vi "BDSCTRL_Read_Configuration_Settings_File.vi"(0 "configuration file path":path, 5 "error in \n(no error)":errorcluster) -> (6 "Channels Cluster":T7={"TX1"=TRUE, "TX2"=TRUE, "TX3"=FALSE, "TX4"=FALSE, "TXx3"=TRUE, "TXx4"=TRUE, "RX1"=FALSE, "RX2"=FALSE, "RX3"=FALSE, "RX4"=FALSE, "RXx3"=FALSE, "RXx4"=FALSE, "Tx"=TRUE, "Rx"=FALSE}, 7 "Set Beam Settings Cluster":T2, 8 "Beam Rotation":string[][](table)=[["1"], ["1"], ["1"], ["1"], ["1"], ["1"], ["2"], ["2"], ["2"], ["2"], ["2"], ["2"]], 9 "DMA Settings Cluster":T1, 10 "Target Devices Settings Cluster":T4={"Target Devices"={"P1 Cluster"={"P1_D1"=TRUE, "P1_D2"=TRUE, "P1_D3"=TRUE, "P1_D4"=TRUE, "P1_D5"=TRUE, "P1_D6"=TRUE, "P1_D7"=TRUE, "P1_D8"=TRUE, "P1_D9"=TRUE, "P1_D10"=TRUE, "P1_D11"=TRUE, "P1_D12"=TRUE, "P1_D13"=TRUE, "P1_D14"=TRUE, "P1_D15"=TRUE, "P1_D16"=TRUE, "P1_D17"=TRUE, "P1_D18"=TRUE, "P1_D19"=TRUE, "P1_D20"=TRUE, "P1_D21"=TRUE, "P1_D22"=TRUE, "P1_D23"=TRUE, "P1_D24"=TRUE}, "P2 Cluster"={"P2_D1"=TRUE, "P2_D2"=TRUE, "P2_D3"=TRUE, "P2_D4"=TRUE, "P2_D5"=TRUE, "P2_D6"=TRUE, "P2_D7"=TRUE, "P2_D8"=TRUE, "P2_D9"=TRUE, "P2_D10"=TRUE, "P2_D11"=TRUE, "P2_D12"=TRUE, "P2_D13"=TRUE, "P2_D14"=TRUE, "P2_D15"=TRUE, "P2_D16"=TRUE, "P2_D17"=TRUE, "P2_D18"=TRUE, "P2_D19"=TRUE, "P2_D20"=TRUE, "P2_D21"=TRUE, "P2_D22"=TRUE, "P2_D23"=TRUE, "P2_D24"=TRUE}}, "Target String"="{1:24,1:24,[],[]}"}, 11 "MB-CFR Settings Cluster":T5, 12 "RF Parameters Settings Cluster":T3={"Tx RF \nFrequency"=2132.5, "RF Bandwidth \n(MHz)"=0, "Tx VGA"=[], "Rx VGA"=[]}, 14 "BDSCTRL Connection Settings":T9={"Panel IP Address"="10.1.11.247", "Melvitron IP Address"="COM12", "EXA IP Address"="10.1.11.123", "MXG IP Address"="10.1.11.122"}, 15 "Test Setup Settings":T8={"IF Calibration File"=path "IFCalExample.csv", "Beam Lookup Table"=path "BeamLookupTableExample.csv", "Test Environment"=enum."Melvitron", "Panel Mode"=enum."CPRI", "Calibration Mode"=0, "Panel Type"=0, "Band"=0, "Tile"=0, "API Drop"=0} {"API Drop" items=["MAY", "JUNE"]; "Tile" items=["HP-C", "HP-B3"]; "Band" items=["AWS", "PCS-A", "PCS-G"]; "Panel Type" items=["Half", "Full", "Quarter"]; "Calibration Mode" items=["Manual", "SemiAuto", "Auto"]}, 16 "Panel Action Sequence":T6[](array[typedef]) items=["Panel Init", "RF Calibration", "Rotate Beam", "Set RF Frequency", "Initial Calibrations", "Channel Enable", "IF Calibration", "Sense Power", "Measure Temperature", "Set RF Power Level", "Run DMA", "Set RF Bandwidth", "Set CFR", "Set Beam"], 19 "error out":errorcluster)   [LabVIEW 2016]
doc: "Illustrates how to read a configuration settings file.\n\nInstructions:\nRun Write Configuration Settings File.vi, located in the file\\config.llb. Then run this VI and select the appropriate configuration settings file to load."
uses:
  BDSCTRL_Controls/BDSCTRL_Panel_Action_List.ctl
  <vilib>/Utility/config.llb/Read Key (String).vi
  <vilib>/Utility/config.llb/Read Key (Path).vi
  <vilib>/Utility/config.llb/Read Key (U32).vi
  <vilib>/Utility/config.llb/Read Key (Boolean).vi
  <vilib>/Utility/config.llb/Read Key (Double).vi
  <vilib>/Utility/config.llb/Read Key (I32).vi
  <vilib>/Utility/config.llb/NI_LVConfig.lvlib
panel:
  out "Instrument Mode Cluster":T10
  out "Array Indexing":string[](array[string])=["A", "B", "C", "D", "E", "F"]
  out "Test Config Size":i32
  out "Test Array Size":i32
  out "Test Array":T11(array[cluster])=[{"Test Module"=0, "Select"=TRUE, "Configure\nParameters"=FALSE}, {"Test Module"=0, "Select"=FALSE, "Configure\nParameters"=FALSE}, {"Test Module"=0, "Select"=FALSE, "Configure\nParameters"=FALSE}, {"Test Module"=0, "Select"=FALSE, "Configure\nParameters"=FALSE}, {"Test Module"=0, "Select"=FALSE, "Configure\nParameters"=FALSE}, {"Test Module"=0, "Select"=FALSE, "Configure\nParameters"=FALSE}, {"Test Module"=0, "Select"=FALSE, "Configure\nParameters"=FALSE}, {"Test Module"=0, "Select"=FALSE, "Configure\nParameters"=FALSE}, {"Test Module"=0, "Select"=FALSE, "Configure\nParameters"=FALSE}, {"Test Module"=0, "Select"=FALSE, "Configure\nParameters"=FALSE}, {"Test Module"=0, "Select"=FALSE, "Configure\nParameters"=FALSE}, {"Test Module"=0, "Select"=FALSE, "Configure\nParameters"=FALSE}, {"Test Module"=0, "Select"=FALSE, "Configure\nParameters"=FALSE}, {"Test Module"=0, "Select"=FALSE, "Configure\nParameters"=FALSE}, {"Test Module"=0, "Select"=FALSE, "Configure\nParameters"=FALSE}, {"Test Module"=0, "Select"=FALSE, "Configure\nParameters"=FALSE}, {"Test Module"=0, "Select"=FALSE, "Configure\nParameters"=FALSE}, {"Test Module"=0, "Select"=FALSE, "Configure\nParameters"=FALSE}, {"Test Module"=0, "Select"=FALSE, "Configure\nParameters"=FALSE}, {"Test Module"=0, "Select"=FALSE, "Configure\nParameters"=FALSE}] {"Test Module" items=["::Select_a_module::", "Dynamic_Range", "EVM_FreqErr_OutputPower_GainFlatness", "RSSI"]}
  # "DMA"
  # "Set Beam"
  # "RF Parameters"
  # "P2"
  # "P1"
  # "MB-CFR"
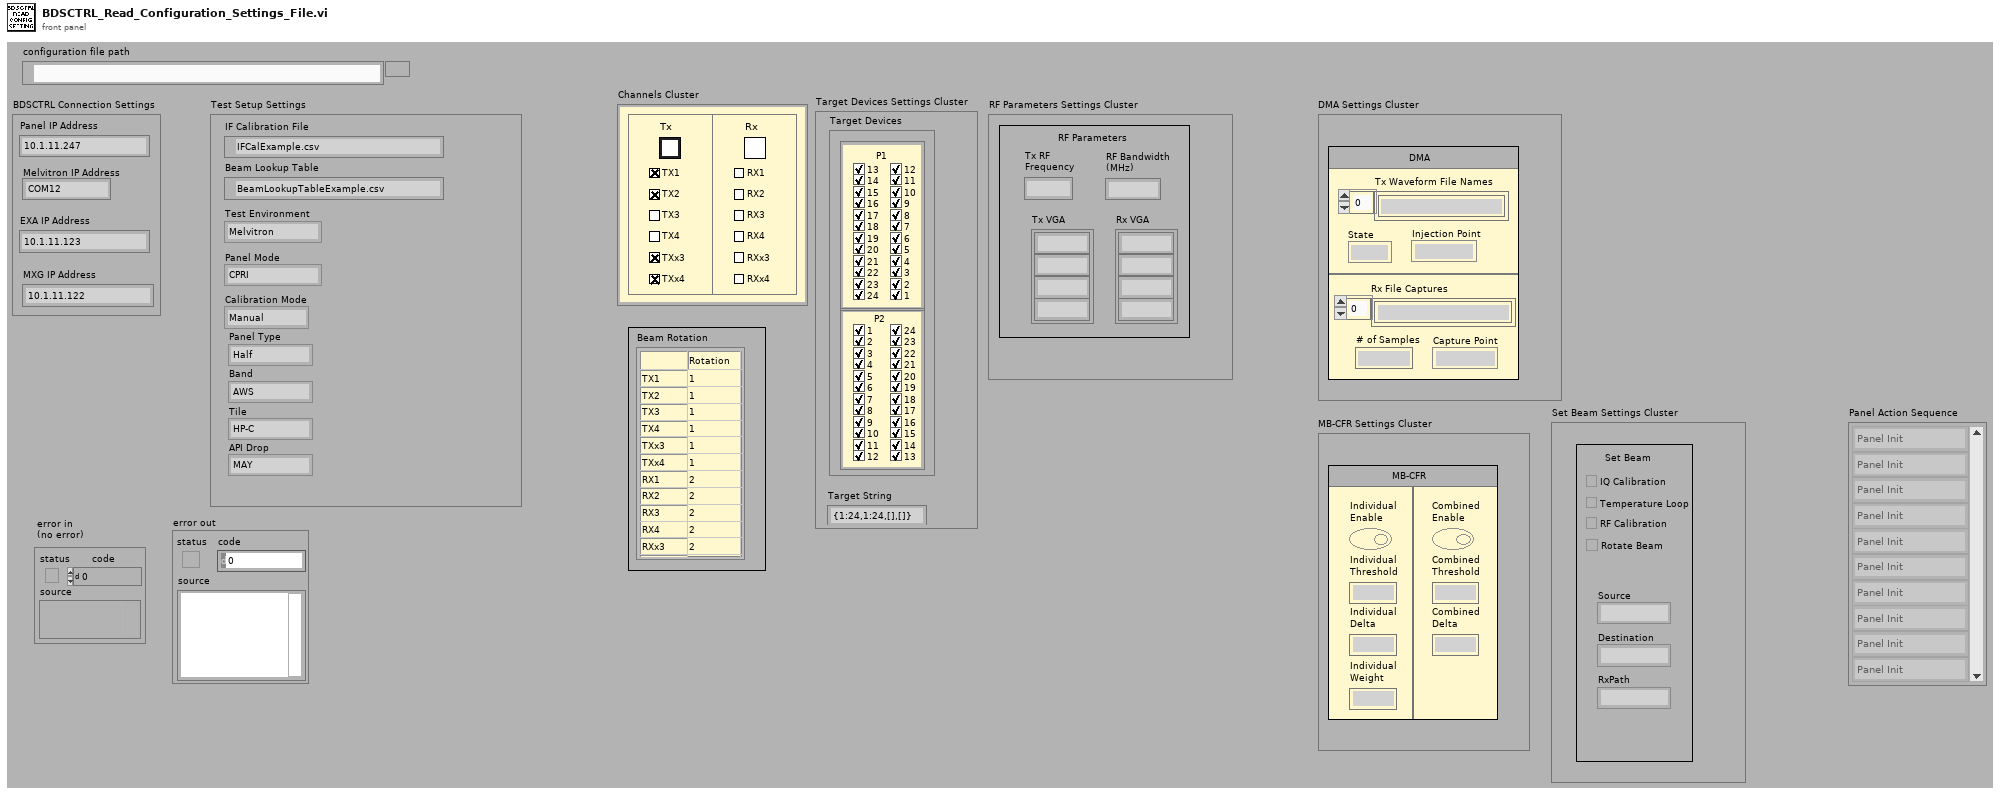
[diagram p1: front panel]
types:
  T1 = cluster{"Tx Waveform File Names":string[], "State":enum16{"Start", "Stop"}, "Injection Point":enum16{"MEM_DAC", "MEM_DUC"}, "Rx File Captures":string[], "# of Samples":i32, "Capture Point":enum16{"MEM_ADC", "MEM_DDC"}}
  T2 = cluster{"IQ Calibration":bool, "Temperature Loop":bool, "RF Calibration":bool, "Rotate Beam":bool, "Source":enum16{"CPRI", "CAL", "MEM_DAC", "MEM_DUC", "EXT"}, "Destination":enum16{"CPRI", "EXT", "MEM_ADC", "MEM_DDC"}, "RxPath":enum16{"DIRECT", "MIXER"}}
  T3 = cluster{"Tx RF \nFrequency":dbl, "RF Bandwidth \n(MHz)":i32, "Tx VGA":i32[], "Rx VGA":i32[]}
  T4 = cluster{"Target Devices":cluster{"P1 Cluster":cluster{"P1_D1":bool, "P1_D2":bool, "P1_D3":bool, "P1_D4":bool, "P1_D5":bool, "P1_D6":bool, "P1_D7":bool, "P1_D8":bool, "P1_D9":bool, "P1_D10":bool, "P1_D11":bool, "P1_D12":bool, "P1_D13":bool, "P1_D14":bool, "P1_D15":bool, "P1_D16":bool, "P1_D17":bool, "P1_D18":bool, "P1_D19":bool, "P1_D20":bool, "P1_D21":bool, "P1_D22":bool, "P1_D23":bool, "P1_D24":bool}, "P2 Cluster":cluster{"P2_D1":bool, "P2_D2":bool, "P2_D3":bool, "P2_D4":bool, "P2_D5":bool, "P2_D6":bool, "P2_D7":bool, "P2_D8":bool, "P2_D9":bool, "P2_D10":bool, "P2_D11":bool, "P2_D12":bool, "P2_D13":bool, "P2_D14":bool, "P2_D15":bool, "P2_D16":bool, "P2_D17":bool, "P2_D18":bool, "P2_D19":bool, "P2_D20":bool, "P2_D21":bool, "P2_D22":bool, "P2_D23":bool, "P2_D24":bool}}, "Target String":string}
  T5 = cluster{"Individual\nEnable":bool, "Individual\nThreshold":dbl, "Individual\nDelta":dbl, "Individual\nWeight":dbl, "Combined\nEnable":bool, "Combined\nThreshold":dbl, "Combined\nDelta":dbl}
  T6 = typedef "BDSCTRL_Panel_Action_List.ctl" = u16
  T7 = cluster{"TX1":bool, "TX2":bool, "TX3":bool, "TX4":bool, "TXx3":bool, "TXx4":bool, "RX1":bool, "RX2":bool, "RX3":bool, "RX4":bool, "RXx3":bool, "RXx4":bool, "Tx":bool, "Rx":bool}
  T8 = cluster{"IF Calibration File":path, "Beam Lookup Table":path, "Test Environment":enum16{"Melvitron", "Spider", "Marinotron"}, "Panel Mode":enum16{"CPRI", "UpDnCnv"}, "Calibration Mode":u16, "Panel Type":u16, "Band":u16, "Tile":u16, "API Drop":u16}
  T9 = cluster{"Panel IP Address":string, "Melvitron IP Address":string, "EXA IP Address":string, "MXG IP Address":string}
  T10 = cluster{"MXA Connection":cluster{"MXA":refnum<visa-resource-name>, "Entry Mode":enum16{"VISA", "IP Address"}}, "MXG1 Connection":cluster{"MXG 1":refnum<visa-resource-name>, "Entry Mode":enum16{"VISA", "IP Address"}}, "MXG2 Connection":cluster{"MXG 2":refnum<visa-resource-name>, "Entry Mode":enum16{"VISA", "IP Address"}}, "MXG3 Connection":cluster{"MXG 3":refnum<visa-resource-name>, "Entry Mode":enum16{"VISA", "IP Address"}}, "ENA Connection":cluster{"ENA":refnum<visa-resource-name>, "Entry Mode":enum16{"VISA", "IP Address"}}}
  T11 = cluster{"Test Module":u16, "Select":bool, "Configure\nParameters":bool}[]
  T12 = typedef "NI_LVConfig.lvlib/Config Data RefNum.ctl" = refnum<k1>
  T13 = cluster{"value":i32, i32[], "value":string, "value":bool, "value":i32, "value":path, "value":path, dbl[][], dbl[][]}
  T14 = cluster{cluster{"value":string, "value":i32}, cluster{"value":string, "value":i32}, cluster{"value":string, "value":i32}, cluster{"value":string, "value":i32}, cluster{"value":string, "value":i32}}
  T15 = cluster{"value":string, "value":string, "value":string, "value":string}
  T16 = cluster{"value":path, "value":path, "value":u32, "value":u32, "value":u32, "value":u32, "value":u32, "value":u32, "value":u32}
  T17 = cluster{"[0]":bool, "[1]":bool, "[2]":bool, "[3]":bool, "[4]":bool, "[5]":bool, "[6]":bool, "[7]":bool, "[8]":bool, "[9]":bool, "[10]":bool, "[11]":bool, "[12]":bool, "[13]":bool}
  T18 = cluster{"[0]":bool, "[1]":bool, "[2]":bool, "[3]":bool, "[4]":bool, "[5]":bool, "[6]":bool, "[7]":bool, "[8]":bool, "[9]":bool, "[10]":bool, "[11]":bool, "[12]":bool, "[13]":bool, "[14]":bool, "[15]":bool, "[16]":bool, "[17]":bool, "[18]":bool, "[19]":bool, "[20]":bool, "[21]":bool, "[22]":bool, "[23]":bool}
  T19 = cluster{"[0]":cluster{"[0]":bool, "[1]":bool, "[2]":bool, "[3]":bool, "[4]":bool, "[5]":bool, "[6]":bool, "[7]":bool, "[8]":bool, "[9]":bool, "[10]":bool, "[11]":bool, "[12]":bool, "[13]":bool, "[14]":bool, "[15]":bool, "[16]":bool, "[17]":bool, "[18]":bool, "[19]":bool, "[20]":bool, "[21]":bool, "[22]":bool, "[23]":bool}, "[1]":cluster{"[0]":bool, "[1]":bool, "[2]":bool, "[3]":bool, "[4]":bool, "[5]":bool, "[6]":bool, "[7]":bool, "[8]":bool, "[9]":bool, "[10]":bool, "[11]":bool, "[12]":bool, "[13]":bool, "[14]":bool, "[15]":bool, "[16]":bool, "[17]":bool, "[18]":bool, "[19]":bool, "[20]":bool, "[21]":bool, "[22]":bool, "[23]":bool}}
  T20 = cluster{cluster{"[0]":cluster{"[0]":bool, "[1]":bool, "[2]":bool, "[3]":bool, "[4]":bool, "[5]":bool, "[6]":bool, "[7]":bool, "[8]":bool, "[9]":bool, "[10]":bool, "[11]":bool, "[12]":bool, "[13]":bool, "[14]":bool, "[15]":bool, "[16]":bool, "[17]":bool, "[18]":bool, "[19]":bool, "[20]":bool, "[21]":bool, "[22]":bool, "[23]":bool}, "[1]":cluster{"[0]":bool, "[1]":bool, "[2]":bool, "[3]":bool, "[4]":bool, "[5]":bool, "[6]":bool, "[7]":bool, "[8]":bool, "[9]":bool, "[10]":bool, "[11]":bool, "[12]":bool, "[13]":bool, "[14]":bool, "[15]":bool, "[16]":bool, "[17]":bool, "[18]":bool, "[19]":bool, "[20]":bool, "[21]":bool, "[22]":bool, "[23]":bool}}, "value":string}
  T21 = cluster{"value":bool, "value":bool, "value":bool, "value":bool, "value":u32, "value":u32, "value":u32}
  T22 = cluster{string[], "value":u32, "value":u32, string[], "value":u32, "value":u32}
  T23 = cluster{"value":bool, "value":dbl, "value":dbl, "value":dbl, "value":bool, "value":dbl, "value":dbl}
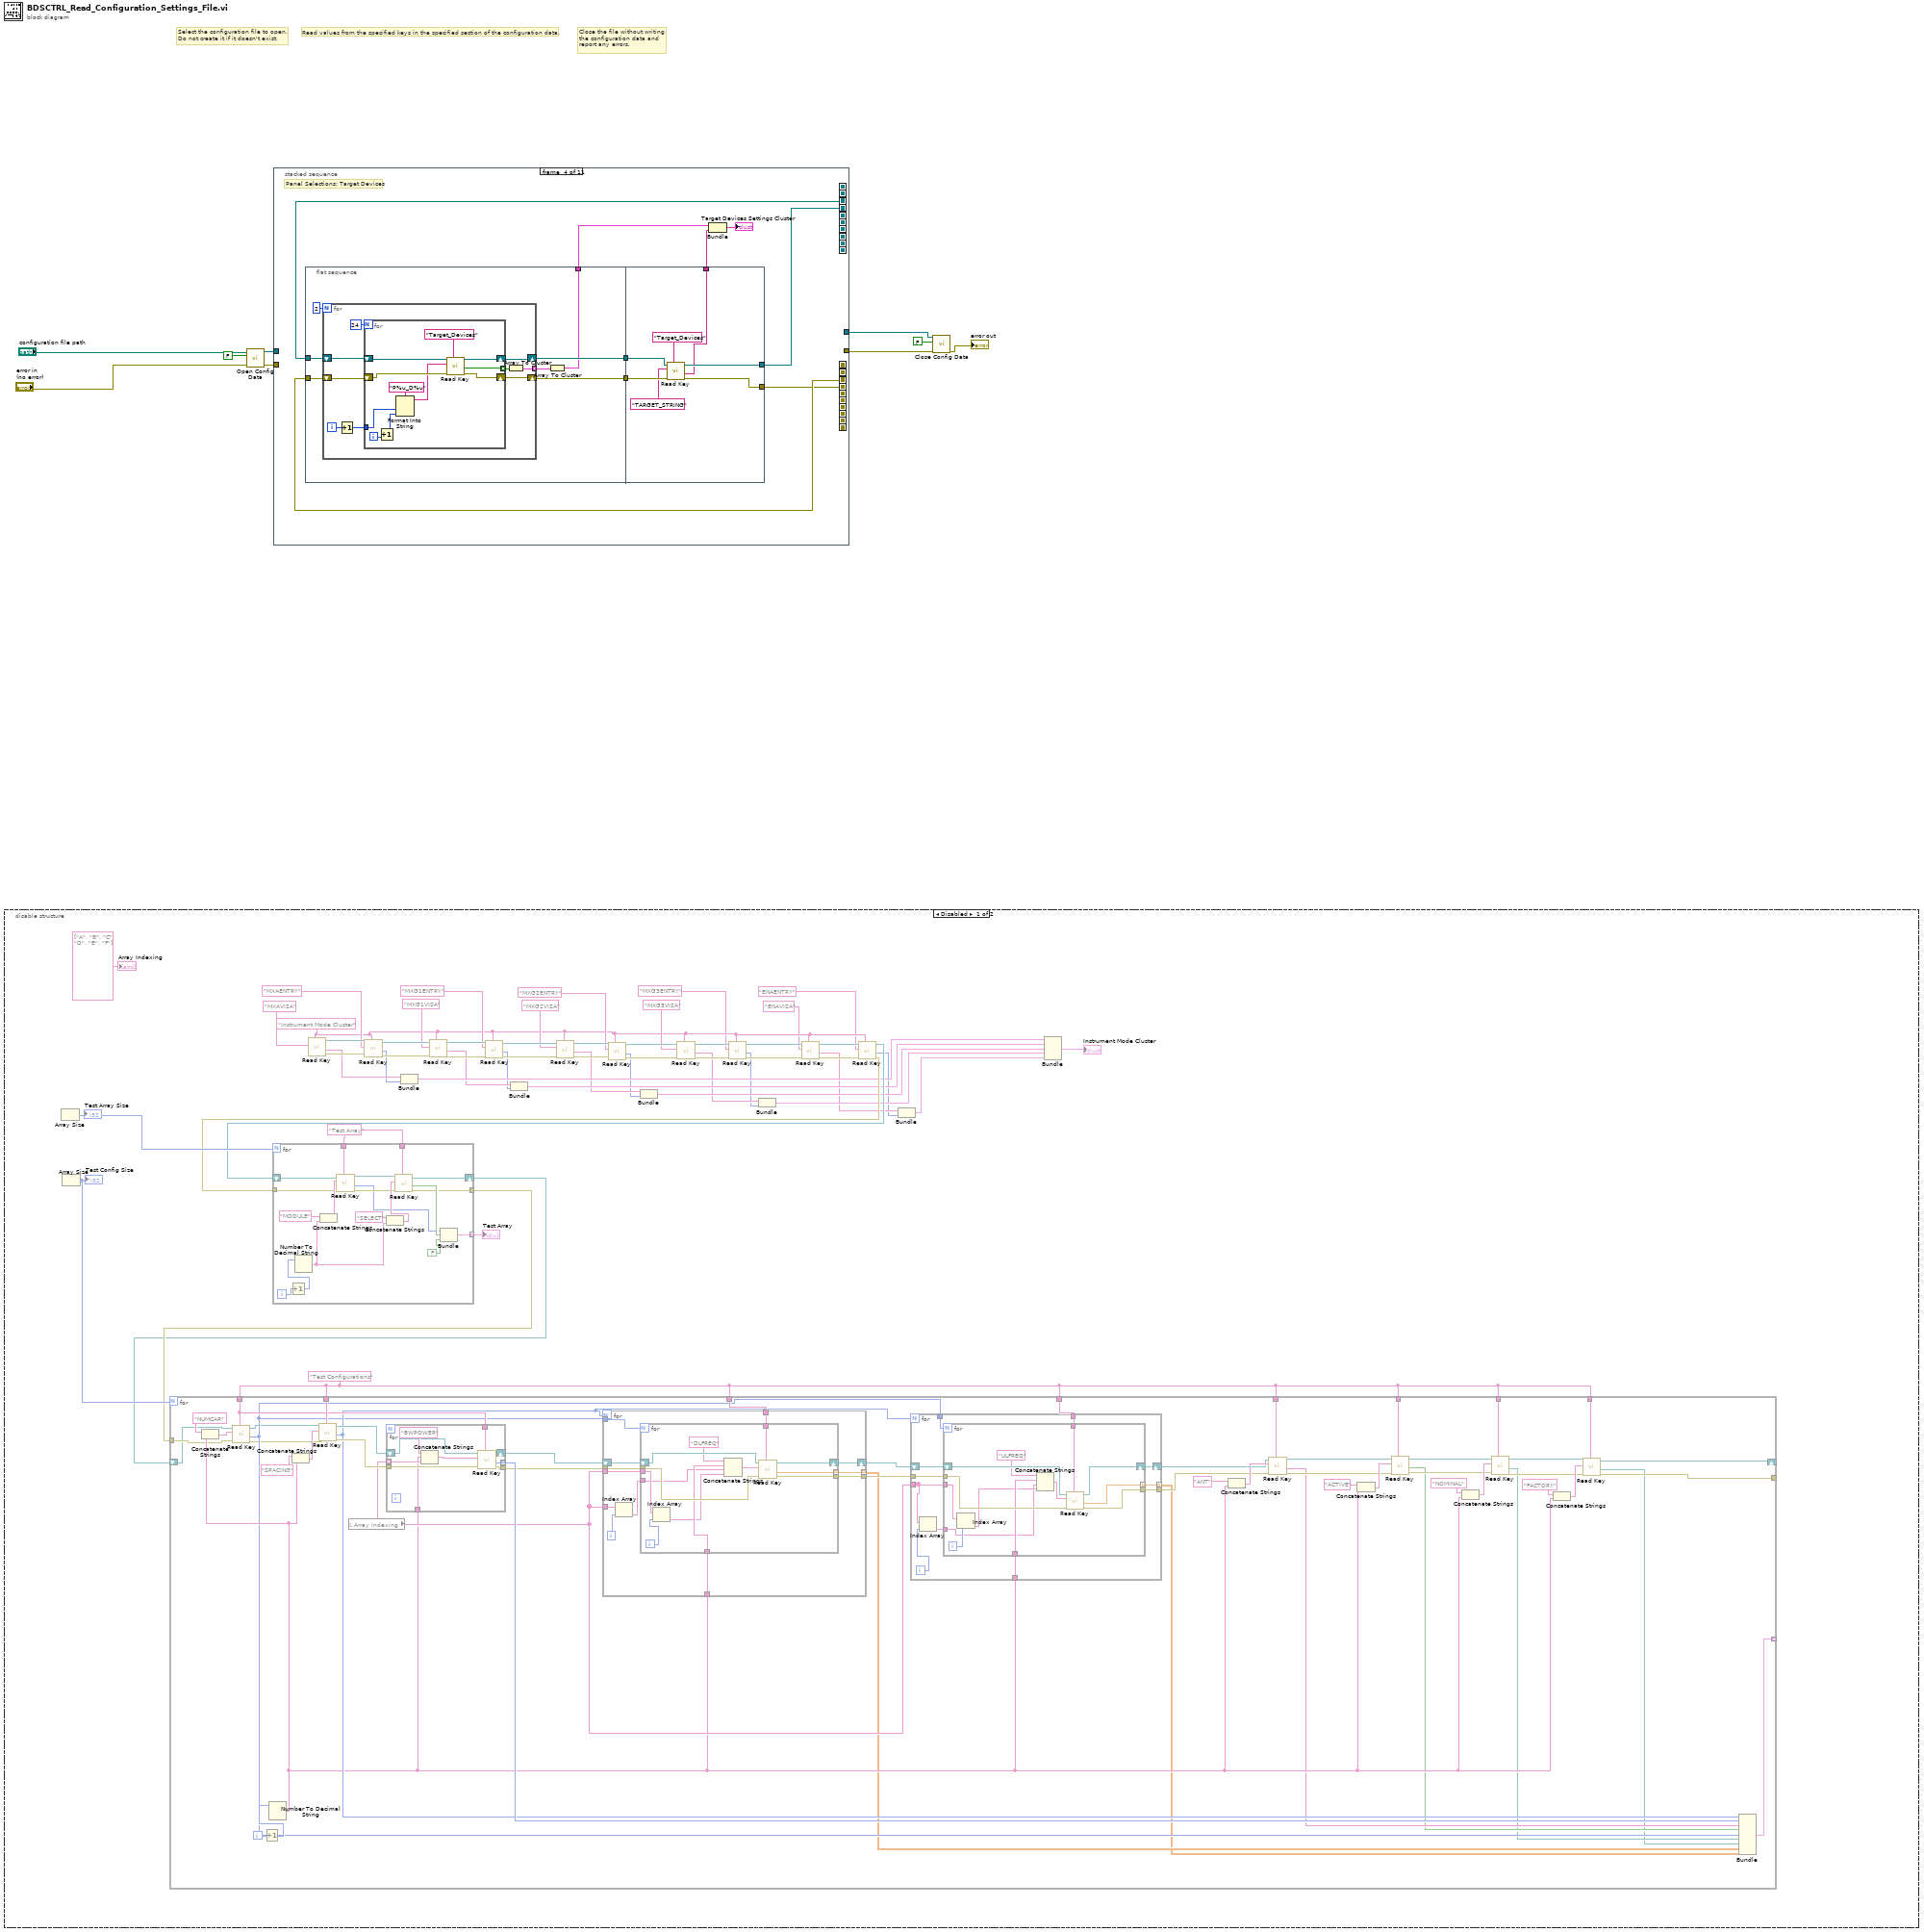
[diagram p0: block diagram]
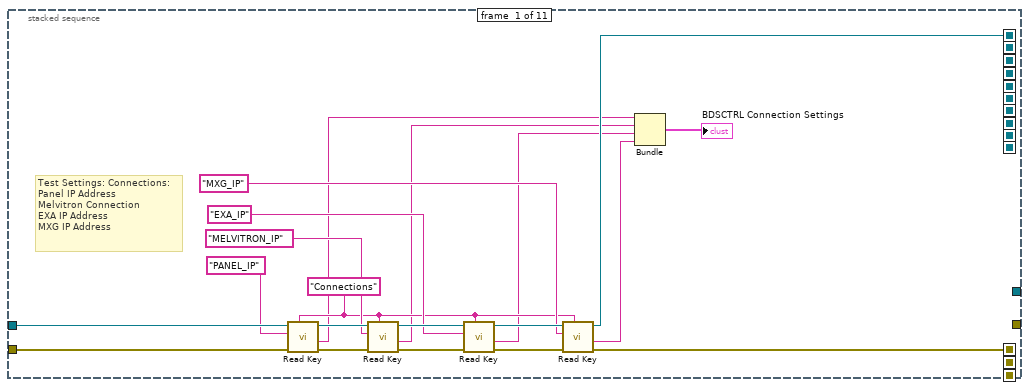
[diagram p3: hidden frame]
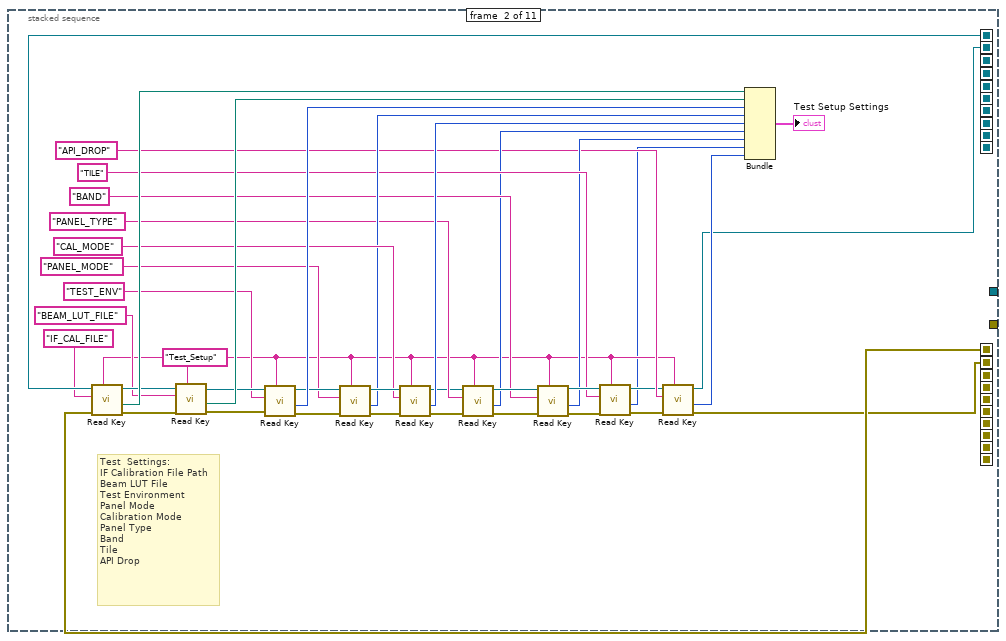
[diagram p4: hidden frame]
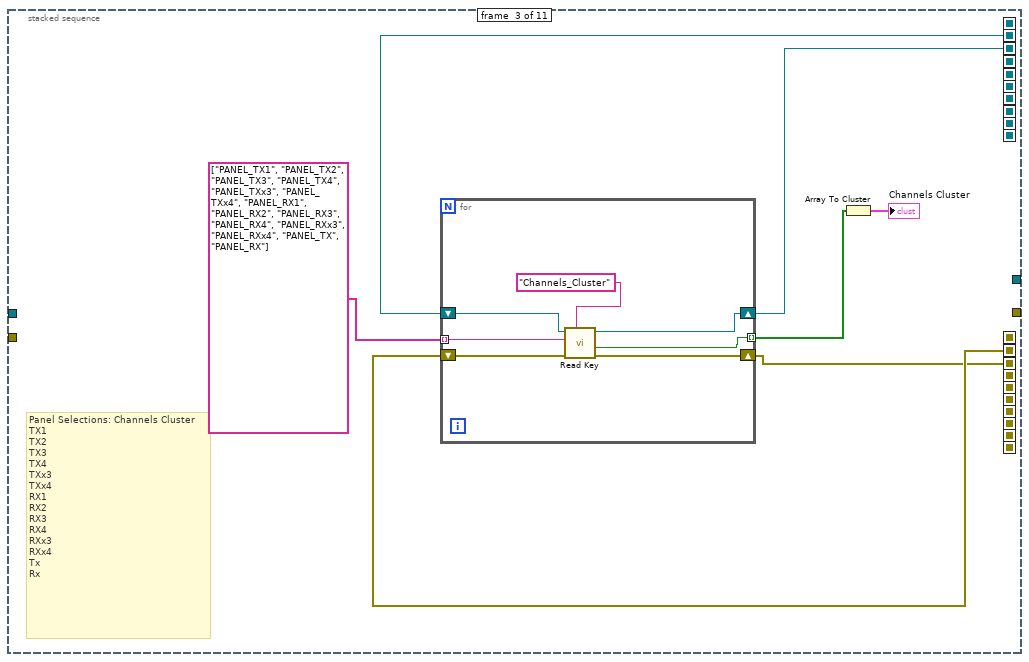
[diagram p5: hidden frame]
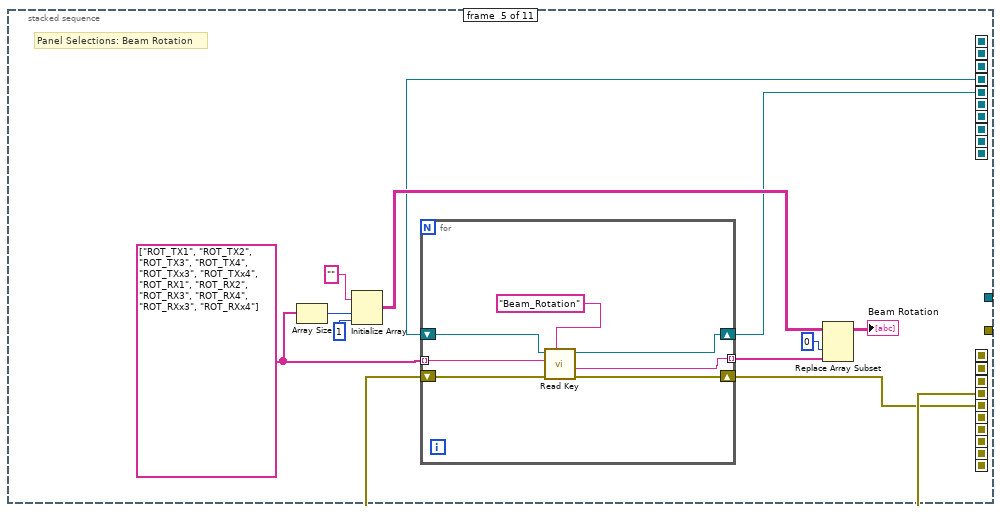
[diagram p6: hidden frame]
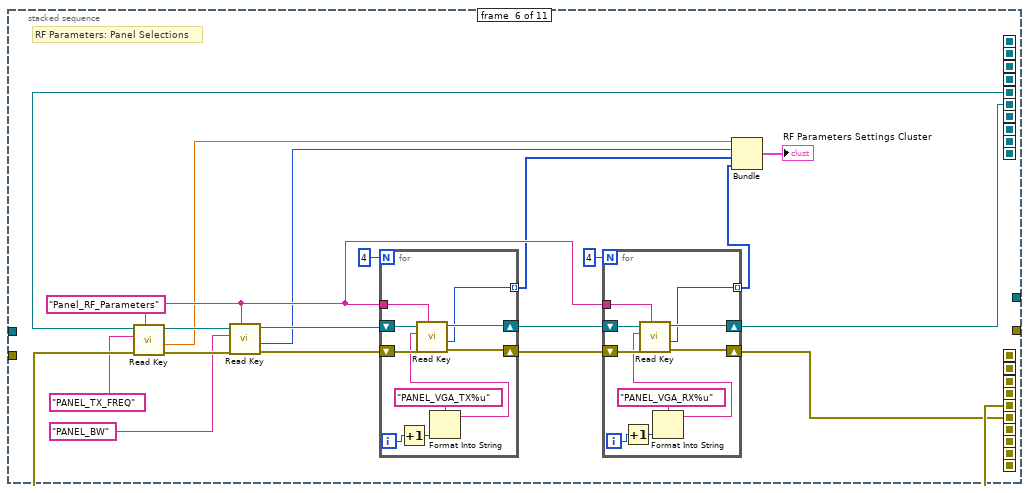
[diagram p7: hidden frame]
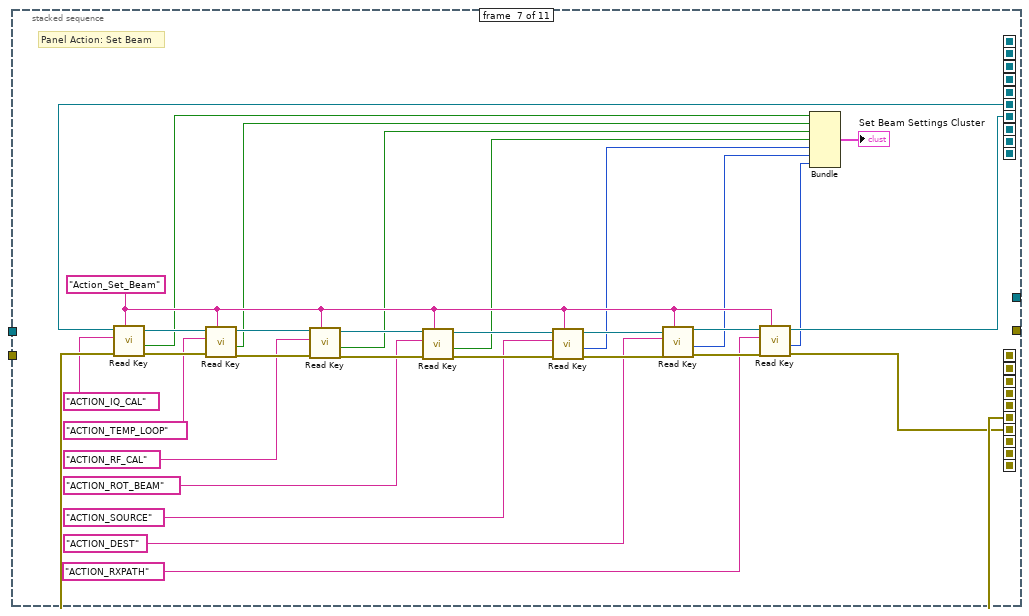
[diagram p8: hidden frame]
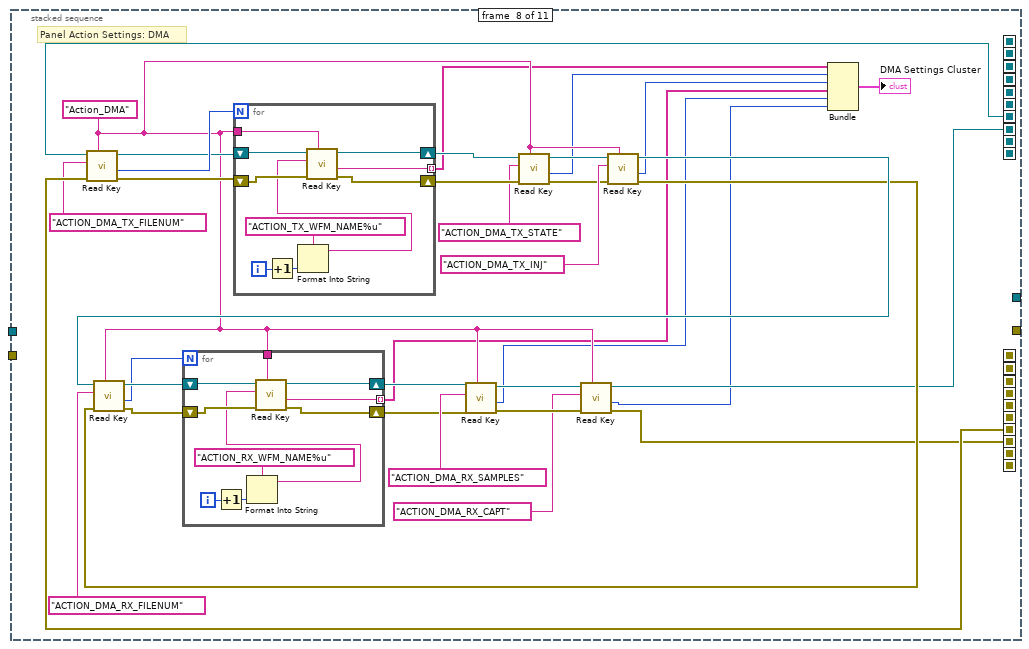
[diagram p9: hidden frame]
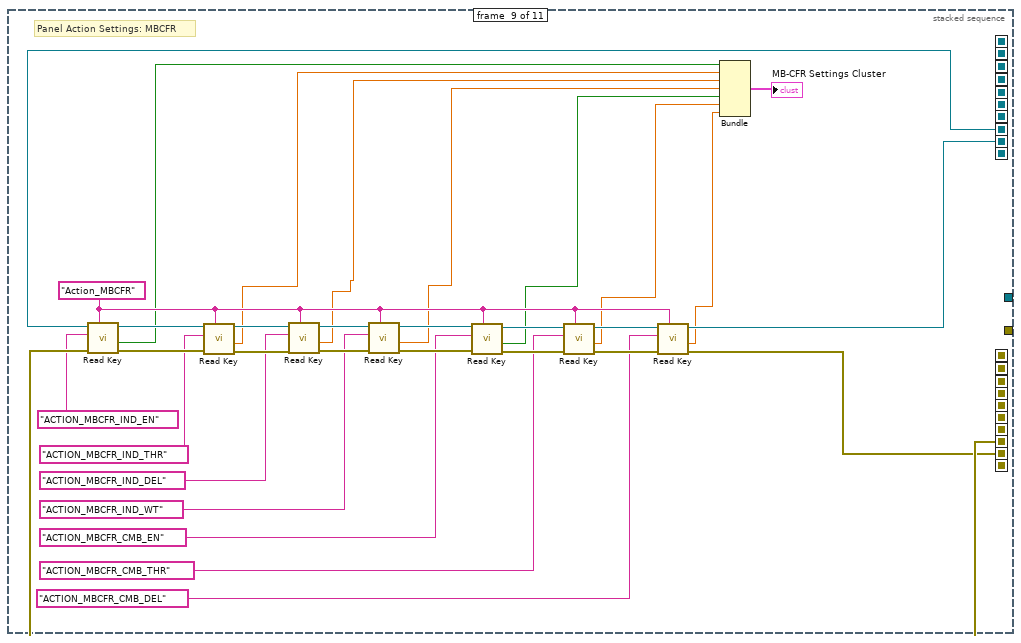
[diagram p10: hidden frame]
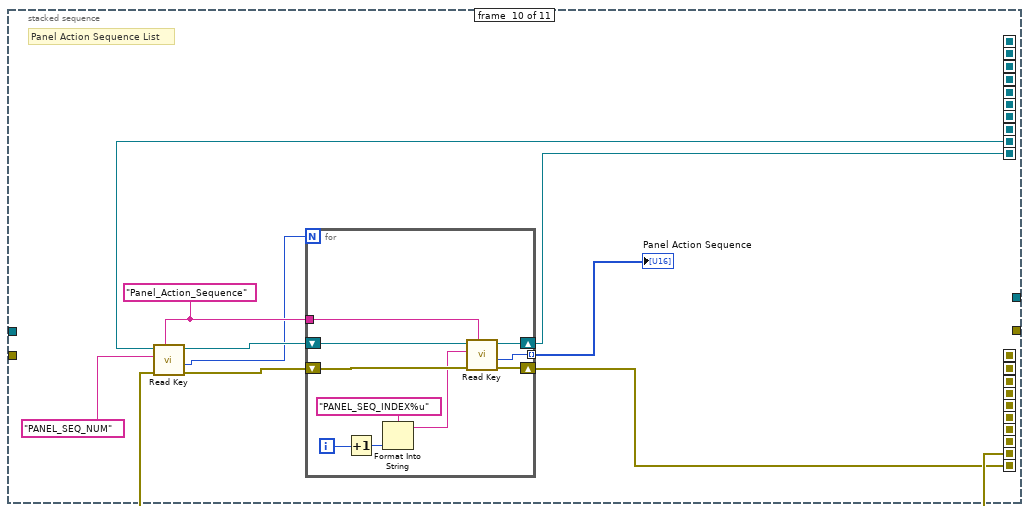
[diagram p11: hidden frame]
diagram:
  # "Close the file without writing\nthe configuration data and\nreport any errors."
  # "Read values from the specified keys in the specified section of the configuration data."
  # "Select the configuration file to open.\nDo not create it if it doesn't exist."
  n1 = disable-structure shown="Disabled" {
    frame Disabled {
      w34 = "Instrument Mode Cluster" ("section")
      w60 = "Test Configurations" ("section")
      w67 = "Test Array" ("section")
      n2 = Array Size() -> (array=w69:dbl[], size(s)=w65:i32)
      "Test Array Size" <- w65
      n3 = Array Size() -> (array=w68:dbl[], size(s)=w64:i32)
      "Test Config Size" <- w64
      n4 = call-poly <vilib>:"Read Key.vi"("section"=w34, "key"="MXAVISA") -> ("error out"=w46:errorcluster, "value"=w26:string, "refnum out"=w58:T12, "error in (no error)"=w47:errorcluster, "refnum"=w59:T12)  [unwired: 4 in, 1 out]
      n5 = call-poly <vilib>:"Read Key.vi"("section"=w34, "error in (no error)"=w46, "key"="MXAENTRY", "refnum"=w58) -> ("error out"=w45:errorcluster, "value"=w25:i32, "refnum out"=w57:T12)  [unwired: 4 in, 1 out]
      n6 = Bundle("value"=w26, "value"=w25) -> (w24:cluster{"value":string, "value":i32})  [unwired: 1 in]
      n7 = call-poly <vilib>:"Read Key.vi"("section"=w34, "error in (no error)"=w45, "key"="MXG1VISA", "refnum"=w57) -> ("error out"=w42:errorcluster, "value"=w23:string, "refnum out"=w56:T12)  [unwired: 4 in, 1 out]
      n8 = call-poly <vilib>:"Read Key.vi"("section"=w34, "error in (no error)"=w42, "key"="MXG1ENTRY", "refnum"=w56) -> ("error out"=w39:errorcluster, "value"=w22:i32, "refnum out"=w55:T12)  [unwired: 4 in, 1 out]
      n9 = Bundle("value"=w23, "value"=w22) -> (w21:cluster{"value":string, "value":i32})  [unwired: 1 in]
      n10 = call-poly <vilib>:"Read Key.vi"("section"=w34, "error in (no error)"=w39, "key"="MXG2VISA", "refnum"=w55) -> ("error out"=w38:errorcluster, "value"=w20:string, "refnum out"=w54:T12)  [unwired: 4 in, 1 out]
      n11 = call-poly <vilib>:"Read Key.vi"("section"=w34, "error in (no error)"=w38, "key"="MXG2ENTRY", "refnum"=w54) -> ("error out"=w36:errorcluster, "value"=w19:i32, "refnum out"=w53:T12)  [unwired: 4 in, 1 out]
      n12 = Bundle("value"=w20, "value"=w19) -> (w18:cluster{"value":string, "value":i32})  [unwired: 1 in]
      n13 = call-poly <vilib>:"Read Key.vi"("section"=w34, "error in (no error)"=w36, "key"="MXG3VISA", "refnum"=w53) -> ("error out"=w35:errorcluster, "value"=w17:string, "refnum out"=w52:T12)  [unwired: 4 in, 1 out]
      n14 = call-poly <vilib>:"Read Key.vi"("section"=w34, "error in (no error)"=w35, "key"="MXG3ENTRY", "refnum"=w52) -> ("error out"=w30:errorcluster, "value"=w16:i32, "refnum out"=w51:T12)  [unwired: 4 in, 1 out]
      n15 = Bundle("value"=w17, "value"=w16) -> (w15:cluster{"value":string, "value":i32})  [unwired: 1 in]
      n16 = call-poly <vilib>:"Read Key.vi"("section"=w34, "error in (no error)"=w30, "key"="ENAVISA", "refnum"=w51) -> ("error out"=w29:errorcluster, "value"=w14:string, "refnum out"=w50:T12)  [unwired: 4 in, 1 out]
      n17 = call-poly <vilib>:"Read Key.vi"("section"=w34, "error in (no error)"=w29, "key"="ENAENTRY", "refnum"=w50) -> ("error out"=w28:errorcluster, "value"=w13:i32, "refnum out"=w27:T12)  [unwired: 4 in, 1 out]
      n18 = for {
        N: w65 -> [_]
        tunnel: w67 -> [w201]
        shift-right: [w184] -> w61
        shift-left: w27 -> [w196]
        tunnel: w28 -> [w195]
        tunnel: w67 -> [w193]
        tunnel: [w188] -> w66 mode=indexing
        tunnel: [w183] -> w63
        i -> [w200]
        n19 = Increment(x=w200) -> (x+1=w199:i32)
        n20 = Number To Decimal String(number=w199) -> (decimal integer string=w191:string)  [unwired: 1 in]
        n21 = Concatenate Strings("MODULE", w191) -> (w197:string)
        n22 = call-poly <vilib>:"Read Key.vi"("section"=w201, "error in (no error)"=w195, "key"=w197, "refnum"=w196) -> ("error out"=w189:errorcluster, "value"=w186:i32, "refnum out"=w194:T12)  [unwired: 4 in, 1 out]
        n23 = Concatenate Strings("SELECT", w191) -> (w190:string)
        n24 = call-poly <vilib>:"Read Key.vi"("section"=w193, "error in (no error)"=w189, "key"=w190, "refnum"=w194) -> ("error out"=w183:errorcluster, "value"=w187:bool, "refnum out"=w184:T12)  [unwired: 4 in, 1 out]
        n25 = Bundle("value"=w186, "value"=w187, FALSE) -> (w188:cluster{"value":i32, "value":bool, bool})  [unwired: 1 in]
      }
      "Test Array" <- w66
      n26 = for {
        N: w64 -> [_]
        tunnel: w63 -> [w75]
        tunnel: w60 -> [w123]
        tunnel: w60 -> [w116]
        tunnel: [w113] -> _ mode=indexing
        tunnel: w60 -> [w110]
        tunnel: w60 -> [w108]
        tunnel: w60 -> [w101]
        tunnel: [w83] -> _
        shift-right: [w84] -> w62
        shift-left: w61 -> [w74]
        tunnel: w60 -> [w99]
        tunnel: w60 -> [w92]
        tunnel: w60 -> [w86]
        i -> [w122]
        n27 = Increment(x=w122) -> (x+1=w121:i32)
        n28 = Number To Decimal String(number=w121) -> (decimal integer string=w85:string)  [unwired: 1 in]
        n29 = Concatenate Strings("NUMCAR", w85) -> (w114:string)
        n30 = call-poly <vilib>:"Read Key.vi"("section"=w99, "error in (no error)"=w75, "key"=w114, "refnum"=w74) -> ("error out"=w70:errorcluster, "value"=w80:i32, "refnum out"=w73:T12)  [unwired: 4 in, 1 out]
        n31 = Concatenate Strings("SPACING", w85) -> (w120:string)
        n32 = call-poly <vilib>:"Read Key.vi"("section"=w123, "error in (no error)"=w70, "key"=w120, "refnum"=w73) -> ("error out"=w111:errorcluster, "value"=w96:i32, "refnum out"=w100:T12)  [unwired: 4 in, 1 out]
        n33 = local read "Array Indexing"() -> (w98:string[])
        n34 = for {
          tunnel: w99 -> [w182]
          tunnel: w111 -> [w181]
          tunnel: [w179] -> w119 mode=indexing
          tunnel: [w178] -> w71
          tunnel: w98 -> [w176] mode=indexing
          tunnel: w85 -> [w174]
          shift-right: [w175] -> w72
          shift-left: w100 -> [w173]
          n35 = Concatenate Strings("BWPOWER", w174, w176) -> (w180:string)
          n36 = call-poly <vilib>:"Read Key.vi"("section"=w182, "error in (no error)"=w181, "key"=w180, "refnum"=w173) -> ("error out"=w178:errorcluster, "value"=w179:i32, "refnum out"=w175:T12)  [unwired: 4 in, 1 out]
        }
        n37 = for {
          N: w96 -> [_]
          tunnel: w110 -> [w159]
          tunnel: w71 -> [w158]
          tunnel: [w157] -> w77 mode=indexing
          tunnel: w98 -> [w156]
          tunnel: [w155] -> w109
          tunnel: w85 -> [w153]
          shift-right: [w154] -> w97
          shift-left: w72 -> [w152]
          tunnel: w80 -> [w151]
          tunnel: w98 -> [w150]
          i -> [w149]
          n38 = Index Array(array=w150, index=w149) -> (element=w148:string)
          n39 = for {
            N: w151 -> [_]
            tunnel: w159 -> [w172]
            tunnel: w158 -> [w171]
            tunnel: [w164] -> w157 mode=indexing
            tunnel: w156 -> [w166]
            tunnel: [w170] -> w155
            tunnel: w153 -> [w168]
            shift-right: [w169] -> w154
            shift-left: w152 -> [w167]
            tunnel: w148 -> [w161]
            i -> [w165]
            n40 = Index Array(array=w166, index=w165) -> (element=w160:string)
            n41 = Concatenate Strings("DLFREQ", w168, w161, w160) -> (w163:string)
            n42 = call-poly <vilib>:"Read Key.vi"("section"=w172, "error in (no error)"=w171, "key"=w163, "refnum"=w167) -> ("error out"=w170:errorcluster, "value"=w164:dbl, "refnum out"=w169:T12)  [unwired: 4 in, 1 out]
          }
        }
        n43 = for {
          N: w96 -> [_]
          tunnel: w109 -> [w134]
          tunnel: w108 -> [w133]
          tunnel: [w132] -> w107
          tunnel: [w130] -> w76 mode=indexing
          tunnel: w85 -> [w129]
          tunnel: w98 -> [w126]
          shift-right: [w131] -> w106
          shift-left: w97 -> [w128]
          tunnel: w80 -> [w124]
          i -> [w127]
          n44 = Index Array(array=w126, index=w127) -> (element=w125:string)
          n45 = for {
            N: w124 -> [_]
            tunnel: w134 -> [w147]
            tunnel: w133 -> [w146]
            tunnel: [w145] -> w132
            tunnel: [w137] -> w130 mode=indexing
            tunnel: w129 -> [w143]
            tunnel: w126 -> [w140]
            shift-right: [w144] -> w131
            shift-left: w128 -> [w142]
            tunnel: w125 -> [w135]
            i -> [w141]
            n46 = Index Array(array=w140, index=w141) -> (element=w136:string)
            n47 = Concatenate Strings("ULFREQ", w143, w135, w136) -> (w139:string)
            n48 = call-poly <vilib>:"Read Key.vi"("section"=w146, "error in (no error)"=w147, "key"=w139, "refnum"=w142) -> ("error out"=w145:errorcluster, "value"=w137:dbl, "refnum out"=w144:T12)  [unwired: 4 in, 1 out]
          }
        }
        n49 = Concatenate Strings("ANT", w85) -> (w117:string)
        n50 = call-poly <vilib>:"Read Key.vi"("section"=w116, "error in (no error)"=w107, "key"=w117, "refnum"=w106) -> ("error out"=w102:errorcluster, "value"=w82:string, "refnum out"=w103:T12)  [unwired: 4 in, 1 out]
        n51 = Concatenate Strings("ACTIVE", w85) -> (w104:string)
        n52 = call-poly <vilib>:"Read Key.vi"("section"=w101, "error in (no error)"=w102, "key"=w104, "refnum"=w103) -> ("error out"=w91:errorcluster, "value"=w81:bool, "refnum out"=w93:T12)  [unwired: 4 in, 1 out]
        n53 = Concatenate Strings("NOMINAL", w85) -> (w95:string)
        n54 = call-poly <vilib>:"Read Key.vi"("section"=w92, "error in (no error)"=w91, "key"=w95, "refnum"=w93) -> ("error out"=w87:errorcluster, "value"=w79:path, "refnum out"=w88:T12)  [unwired: 4 in, 1 out]
        n55 = Concatenate Strings("FACTORY", w85) -> (w89:string)
        n56 = call-poly <vilib>:"Read Key.vi"("section"=w86, "error in (no error)"=w87, "key"=w89, "refnum"=w88) -> ("error out"=w83:errorcluster, "value"=w78:path, "refnum out"=w84:T12)  [unwired: 4 in, 1 out]
        n57 = Bundle("value"=w96, w119, "value"=w82, "value"=w81, "value"=w80, "value"=w79, "value"=w78, w77, w76) -> (w113:T13)  [unwired: 1 in]
      }
      n58 = Bundle("value"=w14, "value"=w13) -> (w12:cluster{"value":string, "value":i32})  [unwired: 1 in]
      n59 = Bundle(w24, w21, w18, w15, w12) -> (→"Instrument Mode Cluster":T14)  [unwired: 1 in]
      "Array Indexing" <- string[] ["A", "B", "C", "D", "E", "F"]
    }
    frame Enabled {
    }
  }
  n60 = call <vilib>:"Open Config Data.vi"("error in (no error)"="error in \n(no error)", "create file if necessary (T)"=FALSE ("create file if necessary? (T)"), "configuration file path"="configuration file path") -> ("error out"=w9:errorcluster, "refnum"=w8:T12)  [unwired: 6 in, 1 out]
  n61 = stacked-sequence {
    seq-local: [w207 _ _ _ _ _ _ _ _ _ _] -> [_ w261 _ _ _ _ _ _ _ _ _]
    seq-local: [w208 _ _ _ _ _ _ _ _ _ _] -> [_ w259 _ _ _ _ _ _ _ _ _]
    seq-local: [_ w223 _ _ _ _ _ _ _ _ _] -> [_ _ w267 _ _ _ _ _ _ _ _]
    seq-local: [_ w222 _ _ _ _ _ _ _ _ _] -> [_ _ w268 _ _ _ _ _ _ _ _]
    seq-local: [_ _ w262 _ _ _ _ _ _ _ _] -> [_ _ _ w284 _ _ _ _ _ _ _]
    seq-local: [_ _ w263 _ _ _ _ _ _ _ _] -> [_ _ _ w283 _ _ _ _ _ _ _]
    seq-local: [_ _ _ w279 _ _ _ _ _ _ _] -> [_ _ _ _ w323 _ _ _ _ _ _]
    seq-local: [_ _ _ w280 _ _ _ _ _ _ _] -> [_ _ _ _ w321 _ _ _ _ _ _]
    seq-local: [_ _ _ _ w322 _ _ _ _ _ _] -> [_ _ _ _ _ w356 _ _ _ _ _]
    seq-local: [_ _ _ _ w320 _ _ _ _ _ _] -> [_ _ _ _ _ w357 _ _ _ _ _]
    seq-local: [_ _ _ _ _ w346 _ _ _ _ _] -> [_ _ _ _ _ _ w409 _ _ _ _]
    seq-local: [_ _ _ _ _ w345 _ _ _ _ _] -> [_ _ _ _ _ _ w408 _ _ _ _]
    seq-local: [_ _ _ _ _ _ w387 _ _ _ _] -> [_ _ _ _ _ _ _ w442 _ _ _]
    seq-local: [_ _ _ _ _ _ w386 _ _ _ _] -> [_ _ _ _ _ _ _ w443 _ _ _]
    seq-local: [_ _ _ _ _ _ _ w418 _ _ _] -> [_ _ _ _ _ _ _ _ w495 _ _]
    seq-local: [_ _ _ _ _ _ _ w417 _ _ _] -> [_ _ _ _ _ _ _ _ w494 _ _]
    seq-local: [_ _ _ _ _ _ _ _ w474 _ _] -> [_ _ _ _ _ _ _ _ _ w504 _]
    seq-local: [_ _ _ _ _ _ _ _ w473 _ _] -> [_ _ _ _ _ _ _ _ _ w501 _]
    seq-local: [_ _ _ _ _ _ _ _ _ w497 _] -> [_ _ _ _ _ _ _ _ _ _ w517]
    seq-local: [_ _ _ _ _ _ _ _ _ w498 _] -> [_ _ _ _ _ _ _ _ _ _ w516]
    tunnel: w9 -> [w219 _ _ _ _ _ _ _ _ _ _]
    tunnel: w8 -> [w218 _ _ _ _ _ _ _ _ _ _]
    tunnel: [_ _ _ _ _ _ _ _ _ _ w517] -> w2
    tunnel: [_ _ _ _ _ _ _ _ _ _ w516] -> w1
    frame #0 {
      w209 = "Connections" ("section")
      # "Test Settings: Connections:\nPanel IP Address\nMelvitron Connection\nEXA IP Address\nMXG IP Address"
      n62 = call-poly <vilib>:"Read Key.vi"("section"=w209, "error in (no error)"=w219, "key"="PANEL_IP", "refnum"=w218) -> ("error out"=w221:errorcluster, "value"=w206:string, "refnum out"=w220:T12)  [unwired: 4 in, 1 out]
      n63 = call-poly <vilib>:"Read Key.vi"("section"=w209, "error in (no error)"=w221, "key"="MELVITRON_IP", "refnum"=w220) -> ("error out"=w216:errorcluster, "value"=w205:string, "refnum out"=w214:T12)  [unwired: 4 in, 1 out]
      n64 = call-poly <vilib>:"Read Key.vi"("section"=w209, "error in (no error)"=w216, "key"="EXA_IP", "refnum"=w214) -> ("error out"=w212:errorcluster, "value"=w204:string, "refnum out"=w211:T12)  [unwired: 4 in, 1 out]
      n65 = call-poly <vilib>:"Read Key.vi"("section"=w209, "error in (no error)"=w212, "key"="MXG_IP", "refnum"=w211) -> ("error out"=w208:errorcluster, "value"=w203:string, "refnum out"=w207:T12)  [unwired: 4 in, 1 out]
      n66 = Bundle("value"=w206, "value"=w205, "value"=w204, "value"=w203) -> (→"BDSCTRL Connection Settings":T15)  [unwired: 1 in]
    }
    frame #1 {
      w227 = "Test_Setup" ("section")
      # "Test  Settings:\nIF Calibration File Path\nBeam LUT File\nTest Environment\nPanel Mode\nCalibration Mode\nPanel Type\nBand\nTile\nAPI Drop"
      n67 = call-poly <vilib>:"Read Key.vi"("section"=w227, "error in (no error)"=w259, "key"="IF_CAL_FILE", "refnum"=w261) -> ("error out"=w256:errorcluster, "value"=w258:path, "refnum out"=w255:T12)  [unwired: 4 in, 1 out]
      n68 = call-poly <vilib>:"Read Key.vi"("section"=w227, "error in (no error)"=w256, "key"="BEAM_LUT_FILE", "refnum"=w255) -> ("error out"=w252:errorcluster, "value"=w253:path, "refnum out"=w250:T12)  [unwired: 4 in, 1 out]
      n69 = call-poly <vilib>:"Read Key.vi"("section"=w227, "error in (no error)"=w252, "key"="TEST_ENV", "refnum"=w250) -> ("error out"=w248:errorcluster, "value"=w251:u32, "refnum out"=w247:T12)  [unwired: 4 in, 1 out]
      n70 = call-poly <vilib>:"Read Key.vi"("section"=w227, "error in (no error)"=w248, "key"="PANEL_MODE", "refnum"=w247) -> ("error out"=w245:errorcluster, "value"=w242:u32, "refnum out"=w244:T12)  [unwired: 4 in, 1 out]
      n71 = call-poly <vilib>:"Read Key.vi"("section"=w227, "error in (no error)"=w245, "key"="CAL_MODE", "refnum"=w244) -> ("error out"=w238:errorcluster, "value"=w241:u32, "refnum out"=w239:T12)  [unwired: 4 in, 1 out]
      n72 = call-poly <vilib>:"Read Key.vi"("section"=w227, "error in (no error)"=w238, "key"="PANEL_TYPE", "refnum"=w239) -> ("error out"=w237:errorcluster, "value"=w231:u32, "refnum out"=w236:T12)  [unwired: 4 in, 1 out]
      n73 = call-poly <vilib>:"Read Key.vi"("section"=w227, "error in (no error)"=w237, "key"="BAND", "refnum"=w236) -> ("error out"=w234:errorcluster, "value"=w230:u32, "refnum out"=w233:T12)  [unwired: 4 in, 1 out]
      n74 = call-poly <vilib>:"Read Key.vi"("section"=w227, "error in (no error)"=w234, "key"="TILE", "refnum"=w233) -> ("error out"=w226:errorcluster, "value"=w225:u32, "refnum out"=w228:T12)  [unwired: 4 in, 1 out]
      n75 = call-poly <vilib>:"Read Key.vi"("section"=w227, "error in (no error)"=w226, "key"="API_DROP", "refnum"=w228) -> ("error out"=w222:errorcluster, "value"=w224:u32, "refnum out"=w223:T12)  [unwired: 4 in, 1 out]
      n76 = Bundle("value"=w258, "value"=w253, "value"=w251, "value"=w242, "value"=w241, "value"=w231, "value"=w230, "value"=w225, "value"=w224) -> (→"Test Setup Settings":T16)  [unwired: 1 in]
    }
    frame #2 {
      # "Panel Selections: Channels Cluster\nTX1\nTX2\nTX3\nTX4\nTXx3\nTXx4\nRX1\nRX2\nRX3\nRX4\nRXx3\nRXx4\nTx\nRx"
      n77 = for {
        shift-right: [w273] -> w263
        shift-left: w268 -> [w274]
        shift-right: [w271] -> w262
        shift-left: w267 -> [w272]
        tunnel: string[] ["PANEL_TX1", "PANEL_TX2", "PANEL_TX3", "PANEL_TX4", "PANEL_TXx3", "PANEL_TXx4", "PANEL_RX1", "PANEL_RX2", "PANEL_RX3", "PANEL_RX4", "PANEL_RXx3", "PANEL_RXx4", "PANEL_TX", "PANEL_RX"] -> [w270] mode=indexing
        tunnel: [w269] -> w264 mode=indexing
        n78 = call-poly <vilib>:"Read Key.vi"("section"="Channels_Cluster", "error in (no error)"=w274, "key"=w270, "refnum"=w272) -> ("error out"=w273:errorcluster, "value"=w269:bool, "refnum out"=w271:T12)  [unwired: 4 in, 1 out]
      }
      n79 = Array To Cluster(array=w264) -> (cluster=→"Channels Cluster":T17)
    }
    frame #3 {
      # "Panel Selections: Target Devices"
      n80 = flat-sequence {
        tunnel: w284 -> [w290]
        tunnel: w283 -> [w289]
        tunnel: [w287] -> w282
        tunnel: [w286] -> w281
        tunnel: [w285] -> w278
        tunnel: w282 -> [w318]
        tunnel: w281 -> [w317]
        tunnel: [w314] -> w280
        tunnel: [w313] -> w279
        tunnel: [w312] -> w277
        frame #0 {
          n81 = for {
            N: 2 -> [_]
            shift-right: [w293] -> w286
            shift-left: w290 -> [w299]
            shift-right: [w292] -> w287
            shift-left: w289 -> [w296]
            tunnel: [w294] -> w288 mode=indexing
            i -> [w298]
            n82 = Increment(x=w298) -> (x+1=w297:i32)
            n83 = for {
              N: 24 -> [_]
              shift-right: [w303] -> w293
              shift-left: w299 -> [w305]
              tunnel: w297 -> [w307]
              shift-right: [w302] -> w292
              shift-left: w296 -> [w306]
              tunnel: [w301] -> w295 mode=indexing
              i -> [w309]
              n84 = Increment(x=w309) -> (x+1=w308:i32)
              n85 = Format Into String(format string="P%u_D%u", w307, w308) -> (resulting string=w304:string)  [unwired: 2 in, 1 out]
              n86 = call-poly <vilib>:"Read Key.vi"("section"="Target_Devices", "error in (no error)"=w306, "key"=w304, "refnum"=w305) -> ("error out"=w302:errorcluster, "value"=w301:bool, "refnum out"=w303:T12)  [unwired: 4 in, 1 out]
            }
            n87 = Array To Cluster(array=w295) -> (cluster=w294:T18)
          }
          n88 = Array To Cluster(array=w288) -> (cluster=w285:T19)
        }
        frame #1 {
          n89 = call-poly <vilib>:"Read Key.vi"("section"="Target_Devices", "error in (no error)"=w318, "key"="TARGET_STRING", "refnum"=w317) -> ("error out"=w314:errorcluster, "value"=w312:string, "refnum out"=w313:T12)  [unwired: 4 in, 1 out]
        }
      }
      n90 = Bundle(w278, "value"=w277) -> (→"Target Devices Settings Cluster":T20)  [unwired: 1 in]
    }
    frame #4 {
      w329 = string[] ["ROT_TX1", "ROT_TX2", "ROT_TX3", "ROT_TX4", "ROT_TXx3", "ROT_TXx4", "ROT_RX1", "ROT_RX2", "ROT_RX3", "ROT_RX4", "ROT_RXx3", "ROT_RXx4"]
      # "Panel Selections: Beam Rotation"
      n91 = Array Size(array=w329) -> (size(s)=w328:i32)
      n92 = Initialize Array("", w328, 1 ("dimension size")) -> (w326:string[][])
      n93 = for {
        shift-right: [w335] -> w320
        shift-left: w321 -> [w336]
        shift-right: [w333] -> w322
        shift-left: w323 -> [w334]
        tunnel: w329 -> [w332] mode=indexing
        tunnel: [w331] -> w325 mode=indexing
        n94 = call-poly <vilib>:"Read Key.vi"("section"="Beam_Rotation", "error in (no error)"=w336, "key"=w332, "refnum"=w334) -> ("error out"=w335:errorcluster, "value"=w331:string, "refnum out"=w333:T12)  [unwired: 4 in, 1 out]
      }
      n95 = Replace Array Subset(array=w326, new element=w325, index (col)=0 ("index (row)")) -> (→"Beam Rotation":string[][])  [unwired: 1 in]
    }
    frame #5 {
      w349 = "Panel_RF_Parameters"
      # "RF Parameters: Panel Selections"
      n96 = call-poly <vilib>:"Read Key.vi"("section"=w349, "error in (no error)"=w357, "key"="PANEL_TX_FREQ", "refnum"=w356) -> ("error out"=w353:errorcluster, "value"=w342:dbl, "refnum out"=w354:T12)  [unwired: 4 in, 1 out]
      n97 = call-poly <vilib>:"Read Key.vi"("section"=w349, "error in (no error)"=w353, "key"="PANEL_BW", "refnum"=w354) -> ("error out"=w350:errorcluster, "value"=w341:i32, "refnum out"=w351:T12)  [unwired: 4 in, 1 out]
      n98 = for {
        N: 4 -> [_]
        shift-right: [w376] -> w348
        shift-left: w351 -> [w377]
        shift-right: [w374] -> w347
        shift-left: w350 -> [w375]
        tunnel: w349 -> [w373]
        tunnel: [w370] -> w340 mode=indexing
        i -> [w369]
        n99 = Increment(x=w369) -> (x+1=w368:i32)
        n100 = Format Into String(format string="PANEL_VGA_TX%u", w368) -> (resulting string=w371:string)  [unwired: 2 in, 1 out]
        n101 = call-poly <vilib>:"Read Key.vi"("section"=w373, "error in (no error)"=w375, "key"=w371, "refnum"=w377) -> ("error out"=w374:errorcluster, "value"=w370:i32, "refnum out"=w376:T12)  [unwired: 4 in, 1 out]
      }
      n102 = for {
        N: 4 -> [_]
        shift-right: [w366] -> w346
        shift-left: w348 -> [w367]
        shift-right: [w364] -> w345
        shift-left: w347 -> [w365]
        tunnel: w349 -> [w363]
        tunnel: [w360] -> w339 mode=indexing
        i -> [w359]
        n103 = Increment(x=w359) -> (x+1=w358:i32)
        n104 = Format Into String(format string="PANEL_VGA_RX%u", w358) -> (resulting string=w361:string)  [unwired: 2 in, 1 out]
        n105 = call-poly <vilib>:"Read Key.vi"("section"=w363, "error in (no error)"=w365, "key"=w361, "refnum"=w367) -> ("error out"=w364:errorcluster, "value"=w360:i32, "refnum out"=w366:T12)  [unwired: 4 in, 1 out]
      }
      n106 = Bundle("value"=w342, "value"=w341, w340, w339) -> (→"RF Parameters Settings Cluster":cluster{"value":dbl, "value":i32, i32[], i32[]})  [unwired: 1 in]
    }
    frame #6 {
      w389 = "Action_Set_Beam"
      # "Panel Action: Set Beam"
      n107 = call-poly <vilib>:"Read Key.vi"("section"=w389, "error in (no error)"=w408, "key"="ACTION_IQ_CAL", "refnum"=w409) -> ("error out"=w406:errorcluster, "value"=w385:bool, "refnum out"=w405:T12)  [unwired: 4 in, 1 out]
      n108 = call-poly <vilib>:"Read Key.vi"("section"=w389, "error in (no error)"=w406, "key"="ACTION_TEMP_LOOP", "refnum"=w405) -> ("error out"=w402:errorcluster, "value"=w384:bool, "refnum out"=w403:T12)  [unwired: 4 in, 1 out]
      n109 = call-poly <vilib>:"Read Key.vi"("section"=w389, "error in (no error)"=w402, "key"="ACTION_RF_CAL", "refnum"=w403) -> ("error out"=w399:errorcluster, "value"=w383:bool, "refnum out"=w400:T12)  [unwired: 4 in, 1 out]
      n110 = call-poly <vilib>:"Read Key.vi"("section"=w389, "error in (no error)"=w399, "key"="ACTION_ROT_BEAM", "refnum"=w400) -> ("error out"=w396:errorcluster, "value"=w382:bool, "refnum out"=w397:T12)  [unwired: 4 in, 1 out]
      n111 = call-poly <vilib>:"Read Key.vi"("section"=w389, "error in (no error)"=w396, "key"="ACTION_SOURCE", "refnum"=w397) -> ("error out"=w394:errorcluster, "value"=w381:u32, "refnum out"=w393:T12)  [unwired: 4 in, 1 out]
      n112 = call-poly <vilib>:"Read Key.vi"("section"=w389, "error in (no error)"=w394, "key"="ACTION_DEST", "refnum"=w393) -> ("error out"=w391:errorcluster, "value"=w380:u32, "refnum out"=w390:T12)  [unwired: 4 in, 1 out]
      n113 = call-poly <vilib>:"Read Key.vi"("section"=w389, "error in (no error)"=w391, "key"="ACTION_RXPATH", "refnum"=w390) -> ("error out"=w386:errorcluster, "value"=w379:u32, "refnum out"=w387:T12)  [unwired: 4 in, 1 out]
      n114 = Bundle("value"=w385, "value"=w384, "value"=w383, "value"=w382, "value"=w381, "value"=w380, "value"=w379) -> (→"Set Beam Settings Cluster":T21)  [unwired: 1 in]
    }
    frame #7 {
      w421 = "Action_DMA"
      # "Panel Action Settings: DMA"
      n115 = call-poly <vilib>:"Read Key.vi"("section"=w421, "error in (no error)"=w443, "key"="ACTION_DMA_TX_FILENUM", "refnum"=w442) -> ("error out"=w439:errorcluster, "value"=w440:i32, "refnum out"=w438:T12)  [unwired: 4 in, 1 out]
      n116 = for {
        N: w440 -> [_]
        shift-right: [w460] -> w436
        shift-left: w439 -> [w463]
        shift-right: [w459] -> w437
        shift-left: w438 -> [w462]
        tunnel: w421 -> [w461]
        tunnel: [w458] -> w416 mode=indexing
        i -> [w455]
        n117 = Increment(x=w455) -> (x+1=w456:i32)
        n118 = Format Into String(format string="ACTION_TX_WFM_NAME%u", w456) -> (resulting string=w454:string)  [unwired: 2 in, 1 out]
        n119 = call-poly <vilib>:"Read Key.vi"("section"=w461, "error in (no error)"=w463, "key"=w454, "refnum"=w462) -> ("error out"=w460:errorcluster, "value"=w458:string, "refnum out"=w459:T12)  [unwired: 4 in, 1 out]
      }
      n120 = call-poly <vilib>:"Read Key.vi"("section"=w421, "error in (no error)"=w436, "key"="ACTION_DMA_TX_STATE", "refnum"=w437) -> ("error out"=w432:errorcluster, "value"=w415:u32, "refnum out"=w434:T12)  [unwired: 4 in, 1 out]
      n121 = call-poly <vilib>:"Read Key.vi"("section"=w421, "error in (no error)"=w432, "key"="ACTION_DMA_TX_INJ", "refnum"=w434) -> ("error out"=w429:errorcluster, "value"=w414:u32, "refnum out"=w431:T12)  [unwired: 4 in, 1 out]
      n122 = call-poly <vilib>:"Read Key.vi"("section"=w421, "error in (no error)"=w429, "key"="ACTION_DMA_RX_FILENUM", "refnum"=w431) -> ("error out"=w427:errorcluster, "value"=w426:i32, "refnum out"=w428:T12)  [unwired: 4 in, 1 out]
      n123 = for {
        N: w426 -> [_]
        shift-right: [w451] -> w423
        shift-left: w427 -> [w453]
        shift-right: [w450] -> w425
        shift-left: w428 -> [w452]
        tunnel: [w449] -> w413 mode=indexing
        tunnel: w421 -> [w444]
        i -> [w446]
        n124 = Increment(x=w446) -> (x+1=w447:i32)
        n125 = Format Into String(format string="ACTION_RX_WFM_NAME%u", w447) -> (resulting string=w445:string)  [unwired: 2 in, 1 out]
        n126 = call-poly <vilib>:"Read Key.vi"("section"=w444, "error in (no error)"=w453, "key"=w445, "refnum"=w452) -> ("error out"=w451:errorcluster, "value"=w449:string, "refnum out"=w450:T12)  [unwired: 4 in, 1 out]
      }
      n127 = call-poly <vilib>:"Read Key.vi"("section"=w421, "error in (no error)"=w423, "key"="ACTION_DMA_RX_SAMPLES", "refnum"=w425) -> ("error out"=w422:errorcluster, "value"=w412:u32, "refnum out"=w420:T12)  [unwired: 4 in, 1 out]
      n128 = call-poly <vilib>:"Read Key.vi"("section"=w421, "error in (no error)"=w422, "key"="ACTION_DMA_RX_CAPT", "refnum"=w420) -> ("error out"=w417:errorcluster, "value"=w411:u32, "refnum out"=w418:T12)  [unwired: 4 in, 1 out]
      n129 = Bundle(w416, "value"=w415, "value"=w414, w413, "value"=w412, "value"=w411) -> (→"DMA Settings Cluster":T22)  [unwired: 1 in]
    }
    frame #8 {
      w476 = "Action_MBCFR"
      # "Panel Action Settings: MBCFR"
      n130 = call-poly <vilib>:"Read Key.vi"("section"=w476, "error in (no error)"=w494, "key"="ACTION_MBCFR_IND_EN", "refnum"=w495) -> ("error out"=w492:errorcluster, "value"=w471:bool, "refnum out"=w491:T12)  [unwired: 4 in, 1 out]
      n131 = call-poly <vilib>:"Read Key.vi"("section"=w476, "error in (no error)"=w492, "key"="ACTION_MBCFR_IND_THR", "refnum"=w491) -> ("error out"=w489:errorcluster, "value"=w470:dbl, "refnum out"=w488:T12)  [unwired: 4 in, 1 out]
      n132 = call-poly <vilib>:"Read Key.vi"("section"=w476, "error in (no error)"=w489, "key"="ACTION_MBCFR_IND_DEL", "refnum"=w488) -> ("error out"=w486:errorcluster, "value"=w469:dbl, "refnum out"=w485:T12)  [unwired: 4 in, 1 out]
      n133 = call-poly <vilib>:"Read Key.vi"("section"=w476, "error in (no error)"=w486, "key"="ACTION_MBCFR_IND_WT", "refnum"=w485) -> ("error out"=w482:errorcluster, "value"=w468:dbl, "refnum out"=w483:T12)  [unwired: 4 in, 1 out]
      n134 = call-poly <vilib>:"Read Key.vi"("section"=w476, "error in (no error)"=w482, "key"="ACTION_MBCFR_CMB_EN", "refnum"=w483) -> ("error out"=w480:errorcluster, "value"=w467:bool, "refnum out"=w481:T12)  [unwired: 4 in, 1 out]
      n135 = call-poly <vilib>:"Read Key.vi"("section"=w476, "error in (no error)"=w480, "key"="ACTION_MBCFR_CMB_THR", "refnum"=w481) -> ("error out"=w478:errorcluster, "value"=w466:dbl, "refnum out"=w477:T12)  [unwired: 4 in, 1 out]
      n136 = call-poly <vilib>:"Read Key.vi"("section"=w476, "error in (no error)"=w478, "key"="ACTION_MBCFR_CMB_DEL", "refnum"=w477) -> ("error out"=w473:errorcluster, "value"=w465:dbl, "refnum out"=w474:T12)  [unwired: 4 in, 1 out]
      n137 = Bundle("value"=w471, "value"=w470, "value"=w469, "value"=w468, "value"=w467, "value"=w466, "value"=w465) -> (→"MB-CFR Settings Cluster":T23)  [unwired: 1 in]
    }
    frame #9 {
      w502 = "Panel_Action_Sequence"
      # "Panel Action Sequence List"
      n138 = call-poly <vilib>:"Read Key.vi"("section"=w502, "error in (no error)"=w501, "key"="PANEL_SEQ_NUM", "refnum"=w504) -> ("error out"=w500:errorcluster, "value"=w496:u32, "refnum out"=w503:T12)  [unwired: 4 in, 1 out]
      n139 = for {
        N: w496 -> [_]
        shift-right: [w508] -> w497
        shift-left: w503 -> [w515]
        shift-right: [w507] -> w498
        shift-left: w500 -> [w513]
        tunnel: w502 -> [w514]
        tunnel: [w506] -> w499 mode=indexing
        i -> [w511]
        n140 = Increment(x=w511) -> (x+1=w510:i32)
        n141 = Format Into String(format string="PANEL_SEQ_INDEX%u", w510) -> (resulting string=w509:string)  [unwired: 2 in, 1 out]
        n142 = call-poly <vilib>:"Read Key.vi"("section"=w514, "error in (no error)"=w513, "key"=w509, "refnum"=w515) -> ("error out"=w507:errorcluster, "value"=w506:u32, "refnum out"=w508:T12)  [unwired: 4 in, 1 out]
      }
      "Panel Action Sequence" <- w499
    }
    frame #10 {
    }
  }
  n143 = call <vilib>:"Close Config Data.vi"("error in (no error)"=w1, "write file if changed (T)"=FALSE ("write configuration file? (T)"), "refnum"=w2) -> ("error out"=→"error out":errorcluster)  [unwired: 8 out]
